vi "linear interpolation - real.vi"(7 "n":i32=-1, 11 "Array":dbl[](array[numeric])) -> (0 "interpolated average":dbl, 1 "mean":dbl, 2 "sum n z_n":dbl, 3 "sum z_n":dbl, 4 "slope":dbl, 6 "intercept":dbl)   [LabVIEW 2016]
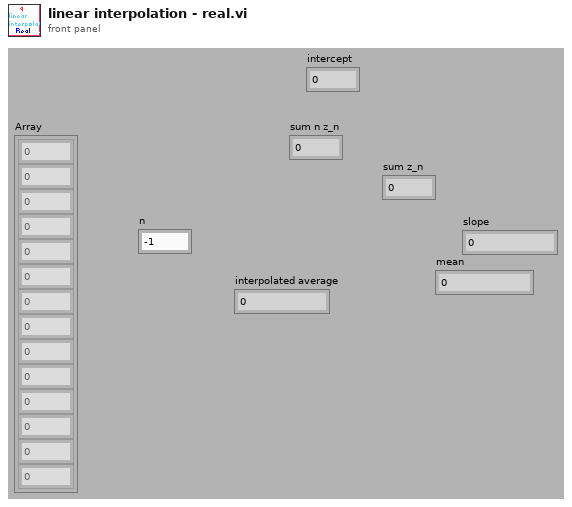
[diagram p1: front panel]
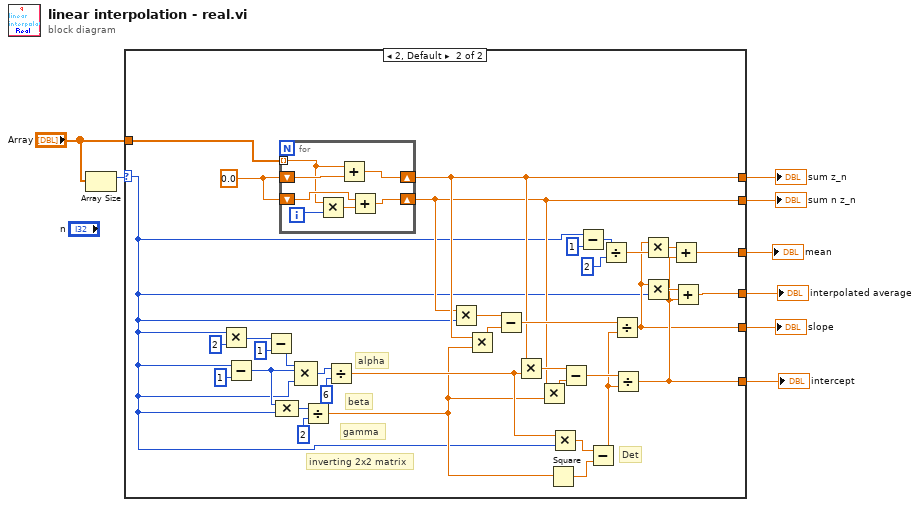
[diagram p0: block diagram]
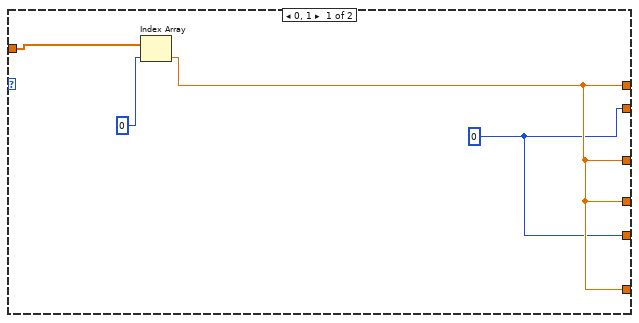
[diagram p2: hidden frame]
diagram:
  n1 = Array Size(array="Array") -> (size(s)=w1:i32)
  n2 = case shown="2, Default" w1 {
    selector: w1 -> [_ w13]
    tunnel: [w10 w20] -> w8
    tunnel: [w9 w19] -> w7
    tunnel: [w10 w18] -> w6
    tunnel: [w10 w17] -> w5
    tunnel: [w10 w16] -> w4
    tunnel: [w9 w15] -> w3
    tunnel: "Array" -> [w12 w14]
    frame 0, 1 {
      w9 = 0 ("index")
      n3 = Index Array(array=w12, index=0) -> (element=w10:dbl)
    }
    frame 2, Default {
      w48 = 0.0
      # "inverting 2x2 matrix"
      # "Det"
      # "beta"
      # "gamma"
      # "alpha"
      n4 = Multiply(x=w13, y=2 ("n")) -> (x*y=w44:i32)
      n5 = Subtract(x=w13, y=1 ("n")) -> (x-y=w40:i32)
      n6 = Subtract(x=w44, y=1 ("n")) -> (x-y=w43:i32)
      n7 = Compound Arithmetic op=MULTIPLY(w40, w13) -> (w38:i32)
      n8 = for {
        tunnel: w14 -> [w49] mode=indexing
        shift-right: [w55] -> w16
        shift-left: w48 -> [w54]
        shift-right: [w52] -> w15
        shift-left: w48 -> [w50]
        i -> [w51]
        n9 = Multiply(x=w49, y=w51) -> (x*y=w53:dbl)
        n10 = Add(x=w49, y=w54) -> (x+y=w55:dbl)
        n11 = Add(x=w50, y=w53) -> (x+y=w52:dbl)
      }
      n12 = Compound Arithmetic op=MULTIPLY(w43, w40, w13) -> (w42:i32)
      n13 = Divide(x=w38, y=2 ("n")) -> (x/y=w29:dbl)
      n14 = Divide(x=w42, y=6 ("n")) -> (x/y=w30:dbl)
      n15 = Multiply(x=w15, y=w13) -> (x*y=w34:dbl)
      n16 = Multiply(x=w16, y=w29) -> (x*y=w35:dbl)
      n17 = Subtract(x=w34, y=w35) -> (x-y=w33:dbl)
      n18 = Multiply(x=w16, y=w30) -> (x*y=w31:dbl)
      n19 = Multiply(x=w15, y=w29) -> (x*y=w32:dbl)
      n20 = Square(x=w29) -> (x^2=w36:dbl)
      n21 = Multiply(x=w30, y=w13) -> (x*y=w37:dbl)
      n22 = Subtract(x=w31, y=w32) -> (x-y=w28:dbl)
      n23 = Subtract(x=w13, y=1 ("n")) -> (x-y=w25:i32)
      n24 = Subtract(x=w37, y=w36) -> (x-y=w27:dbl)
      n25 = Divide(x=w25, y=2 ("n")) -> (x/y=w23:dbl)
      n26 = Divide(x=w33, y=w27) -> (x/y=w19:dbl)
      n27 = Divide(x=w28, y=w27) -> (x/y=w20:dbl)
      n28 = Multiply(x=w19, y=w23) -> (x*y=w22:dbl)
      n29 = Multiply(x=w19, y=w13) -> (x*y=w21:dbl)
      n30 = Add(x=w22, y=w20) -> (x+y=w17:dbl)
      n31 = Add(x=w21, y=w20) -> (x+y=w18:dbl)
    }
  }
  "interpolated average" <- w6
  "slope" <- w7
  "mean" <- w5
  "intercept" <- w8
  "sum n z_n" <- w3
  "sum z_n" <- w4
